vi "Calibrated CMN-SRD-1000_reader.vi"() -> ()   [LabVIEW 2017]
panel:
  in  "SRD-1000":dbl
  out "SRD high limit":dbl
  out "SRD low limit":dbl
  in  "?":bool
  out "CMN-Temperature":dbl
  in  "CMN-1000":dbl
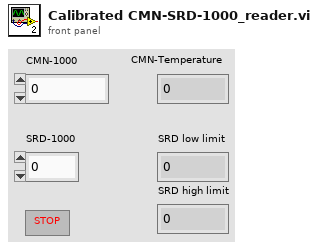
[diagram p1: front panel]
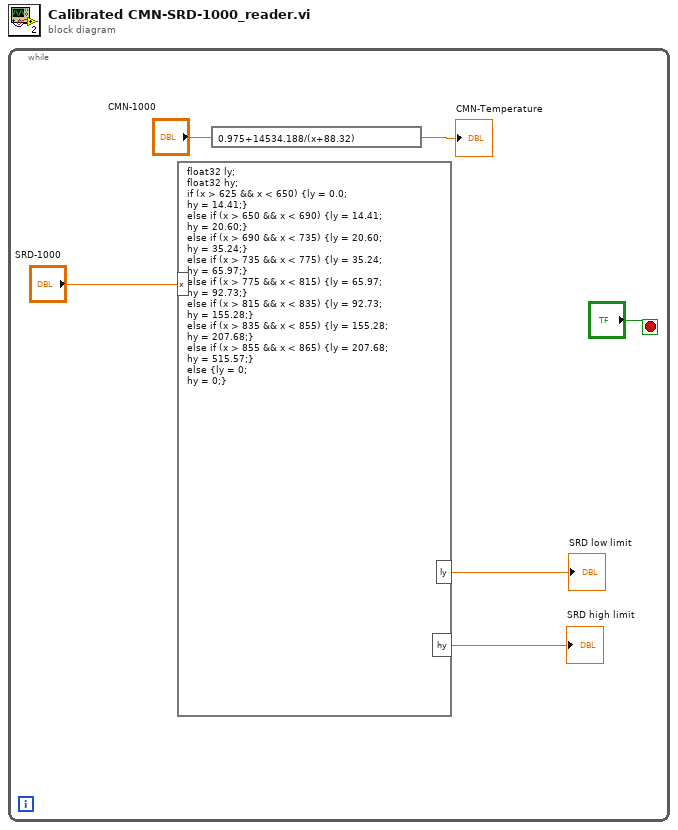
[diagram p0: block diagram]
diagram:
  n1 = while {
    stop <- "?" stop-if-true
    n2 = formula code="float32 ly;\nfloat32 hy;\nif (x > 625 && x < 650) {ly = 0.0;\nhy = 14.41;}\nelse if (x > 650 && x < 690) {ly = 14.41;\nhy = 20.60;}\nelse if (x > 690 && x < 735) {ly = 20.60;\nhy = 35.24;}\nelse if (x > 735 && x < 775) {ly = 35.24;\nhy = 65.97;}\nelse if (x > 775 && x < 815) {ly = 65.97;\nhy = 92.73;}\nelse if (x > 815 && x < 835) {ly = 92.73;\nhy = 155.28;}\nelse if (x > 835 && x < 855) {ly = 155.28;\nhy = 207.68;}\nelse if (x > 855 && x < 865) {ly = 207.68;\nhy = 515.57;}\nelse {ly = 0;\nhy = 0;}"("x"="SRD-1000") -> ("ly"=→"SRD low limit":sgl, "hy"=→"SRD high limit":sgl)
    n3 = expression code="0.975+14534.188/(x+88.32)"("CMN-1000") -> (→"CMN-Temperature":dbl)
  }
